vi "CameraSetting_MainScreen.vi"() -> ()   [LabVIEW 2015]
panel:
  in  "相机高级参数":bool
  in  "设置默认相机":string(combo)
  in  "主页按钮":bool
  in  "保存按钮":bool
  out "当前默认使用相机":string
  in  "相机类型":u16(ring) items=["本地相机", "网络相机"]
  out "相机基本参数":enum32{"本地相机", "网络相机"}(tab)
  out "本地相机参数":string[][](table)
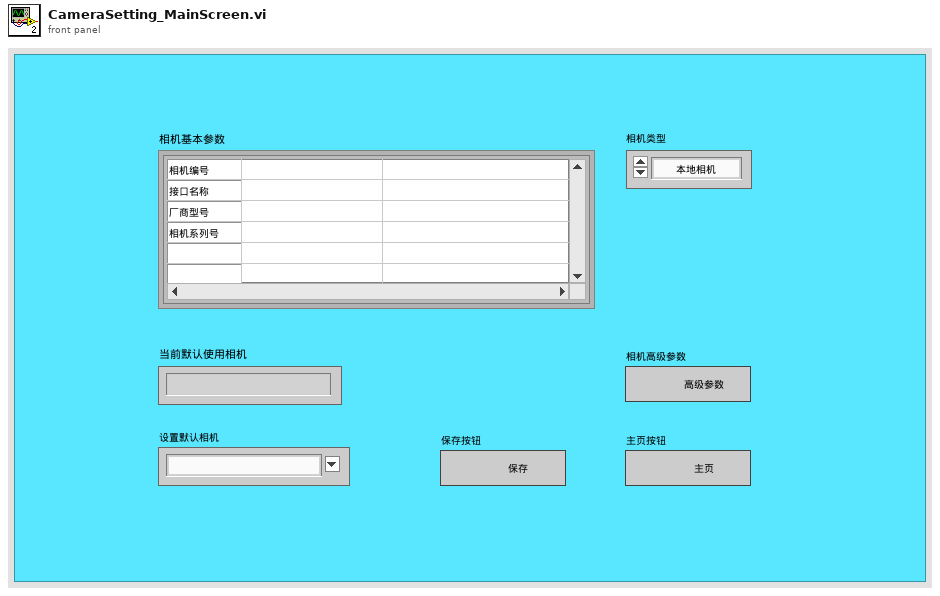
[diagram p1: front panel]
types:
  T1 = enum16{"Boolean", "DBL", "I32", "Path", "String", "U32"}
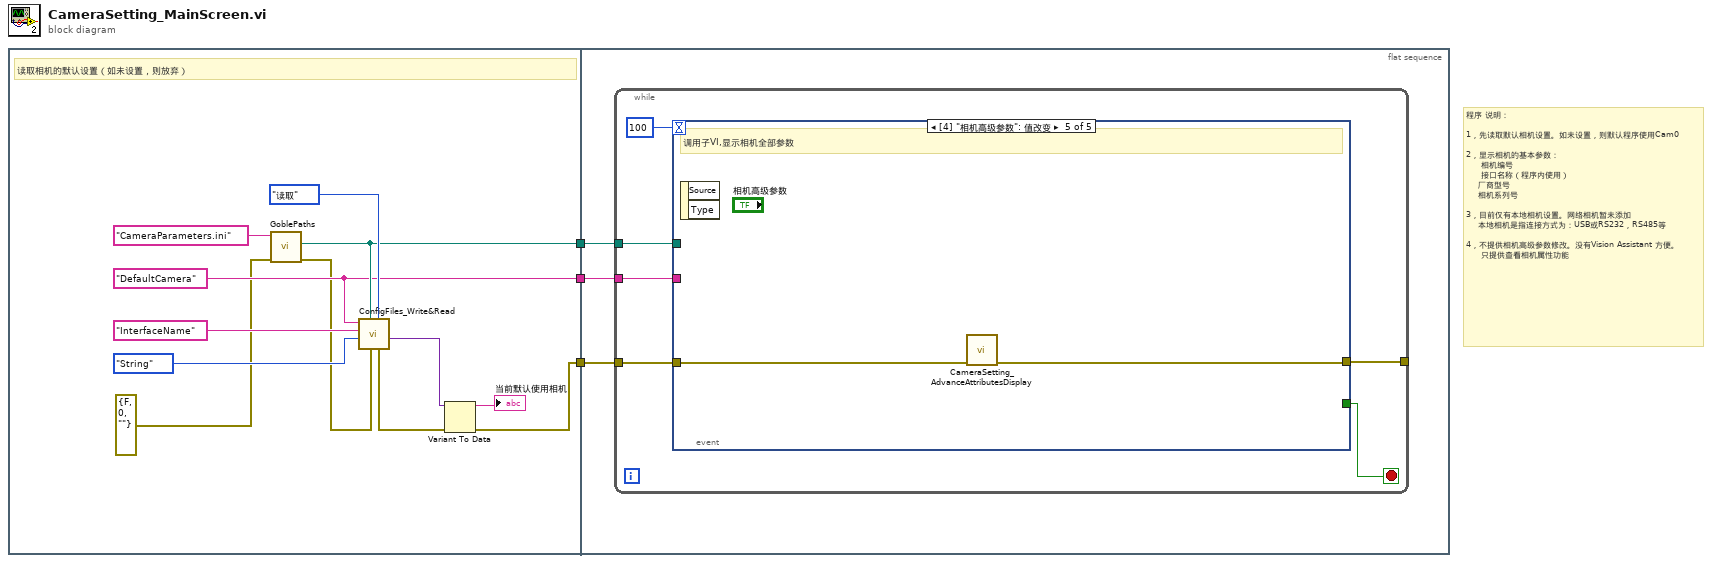
[diagram p0: block diagram]
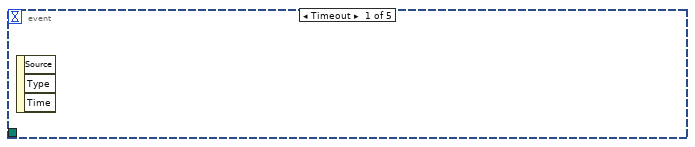
[diagram p2: hidden frame]
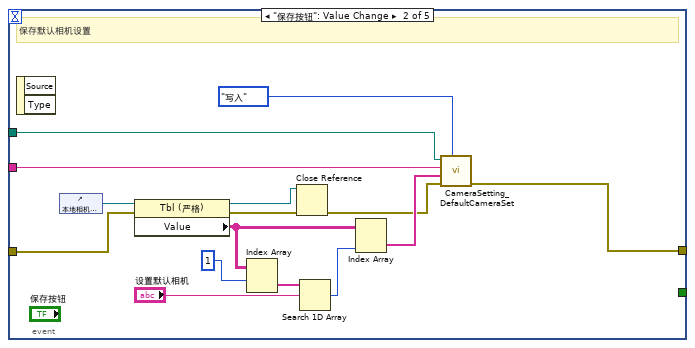
[diagram p3: hidden frame]
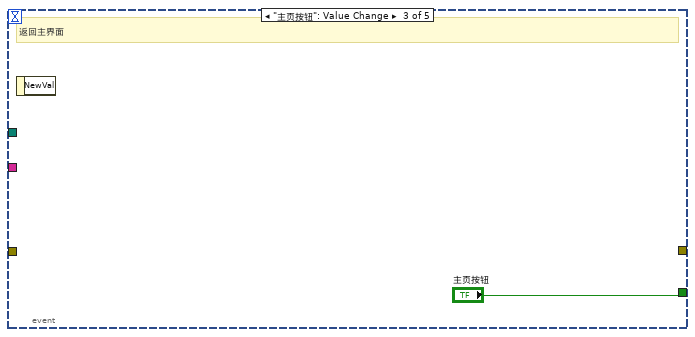
[diagram p4: hidden frame]
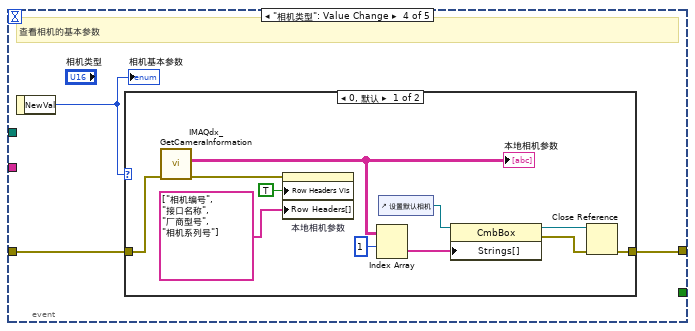
[diagram p5: hidden frame]
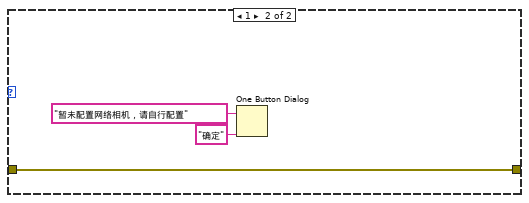
[diagram p6: hidden frame]
diagram:
  # "程序 说明：\n\n1，先读取默认相机设置。如未设置，则默认程序使用Cam0\n\n2，显示相机的基本参数：\n     相机编号 \n     接口名称（程序内使用）\n    厂商型号\n    相机系列号\n\n3，目前仅有本地相机设置。网络相机暂未添加\n    本地相机是指连接方式为：USB或RS232，RS485等\n\n4，不提供相机高级参数修改。没有Vision Assistant 方便。\n     只提供查看相机属性功能"
  n1 = flat-sequence {
    tunnel: [w8] -> w3
    tunnel: [w7] -> w2
    tunnel: [w6] -> w1
    tunnel: w3 -> [w18]
    tunnel: w2 -> [w17]
    tunnel: w1 -> [w16]
    frame #0 {
      w7 = "DefaultCamera" ("字段名称")
      # "读取相机的默认设置（如未设置，则放弃）"
      n2 = call "GoblePaths.vi"("error in (no error)"=errorcluster {"status"=FALSE, "code"=0, "source"=""}, "文件名称"="CameraParameters.ini" ("configuration file path")) -> ("error out"=w4:errorcluster, "文件完整路径"=w8:path)  [unwired: 7 in, 1 out]
      n3 = call "ConfigFiles_Write&Read.vi"("功能类型"=enum16{"读取", "写入"}."读取", "error in (no error)"=w4, "configuration file path"=w8, "键值类型"=T1."String", "键名称"="InterfaceName" ("字段名称"), "字段名称"=w7) -> ("键值_输出"=w12:variant, "error out"=w10:errorcluster)  [unwired: 2 in, 2 out]
      n4 = Variant To Data(error in=w10, Variant=w12) -> (data=→"当前默认使用相机":string, error out=w6:errorcluster)  [unwired: 1 in]
    }
    frame #1 {
      n5 = while {
        tunnel: w18 -> [w22]
        tunnel: w17 -> [w21]
        tunnel: w16 -> [w20]
        tunnel: [w19] -> _
        stop <- w24 stop-if-true
        n6 = event shown="[4] \"相机高级参数\": 值改变" {
          selector: _ -> [_ _ _ _ _]
          dyn-events: _ -> [_ _ _ _ _]
          timeout: 100 -> [_ _ _ _ _]
          tunnel: [_ _ "主页按钮" _ _] -> w24
          tunnel: w22 -> [_ w31 _ _ _]
          tunnel: w21 -> [_ w30 _ _ _]
          tunnel: w20 -> [_ w29 _ w42 w59]
          tunnel: [_ w25 _ w41 w58] -> w19
          event Timeout {
            n7 = event-data() -> ()  [unwired: 1 in, 3 out]
          }
          event "保存按钮": Value Change {
            # "保存默认相机设置"
            n8 = event-data() -> ()  [unwired: 1 in, 2 out]
            n9 = control-ref of="本地相机参数"() -> (w38:refnum<vi>)
            n10 = property class="Tbl (严格)"(reference=w38, error in=w29) -> (reference out=w28:refnum<vi>, error out=w27:errorcluster, "Value"=w34:string[][])
            n11 = Index Array(array=w34, index (row)=1 ("索引 (行)")) -> (element=w37:string[])  [unwired: 1 in]
            n12 = Close Reference(reference=w28, error in (no error)=w27) -> (error out=w26:errorcluster)
            n13 = Search 1D Array(1D array=w37, element="设置默认相机") -> (index of element=w35:i32)  [unwired: 1 in]
            n14 = Index Array(array=w34, index (col)=w35) -> (element=w32:string[])  [unwired: 1 in]
            n15 = call "CameraSetting_DefaultCameraSet.vi"("功能类型"=enum16{"读取", "写入"}."写入", "error in (no error)"=w26, "CameraBasicInfor"=w32, "字段名称"=w30, "configuration file path"=w31) -> ("error out"=w25:errorcluster)  [unwired: 6 in]
          }
          event "主页按钮": Value Change {
            # "返回主界面"
            n16 = event-data() -> ()  [unwired: 1 in, 1 out]
          }
          event "相机类型": Value Change {
            # "查看相机的基本参数"
            n17 = event-data() -> ("NewVal"=w43:u16)  [unwired: 1 in]
            "相机基本参数" <- w43
            n18 = case shown="0, 默认" w43 {
              tunnel: w42 -> [w45 w55]
              tunnel: [w44 w55] -> w41
              frame 0, Default {
                n19 = call "IMAQdx_GetCameraInformation.vi"("error in (no error)"=w45) -> ("error out"=w54:errorcluster, "Camera Basic Information"=w50:string[][])  [unwired: 8 in, 1 out]
                "本地相机参数" <- w50
                n20 = property on="本地相机参数" class="Tbl (严格)"(error in=w54, "Row Headers Vis"=TRUE ("显示项:显示行首"), "Row Headers[]"=string[] ["相机编号", "接口名称", "厂商型号", "相机系列号"]) -> ()  [unwired: 1 in, 2 out]
                n21 = Index Array(array=w50, index (row)=1 ("索引 (行)")) -> (element=w48:string[])  [unwired: 1 in]
                n22 = control-ref of="设置默认相机"() -> (w49:refnum<vi>)
                n23 = property class="CmbBox"(reference=w49, "Strings[]"=w48) -> (reference out=w47:refnum<vi>, error out=w46:errorcluster)  [unwired: 1 in]
                n24 = Close Reference(reference=w47, error in (no error)=w46) -> (error out=w44:errorcluster)
              }
              frame 1 {
                n25 = One Button Dialog(message="暂未配置网络相机，请自行配置" ("消息"), button name ("OK")="确定" ("按钮名称（“确定”）")) -> ()  [unwired: 1 out]
              }
            }
          }
          event "相机高级参数": Value Change {
            # "调用子VI,显示相机全部参数"
            n26 = event-data() -> ()  [unwired: 1 in, 2 out]
            n27 = call "CameraSetting_AdvanceAttributesDisplay.vi"("error in (no error)"=w59) -> ("error out"=w58:errorcluster)  [unwired: 10 in]
          }
        }
      }
    }
  }
